vi "Accumulate data.vi"(6 "block size":i32, 9 "reset":bool, 10 "zero":bool, 11 "Accelerometer Data":T1={"Accel"=[0.0, 0.0, 0.0], "Gyro"=[0.0, 0.0, 0.0], "Time"=0, "Trigger"=FALSE}) -> (1 "done":bool, 2 "number in block":i32, 3 "Accelerometer Data Block":T2)   [LabVIEW 2013]
uses:
  I2C/Accelerometer Data Block.ctl
  I2C/Accelerometer Data.ctl
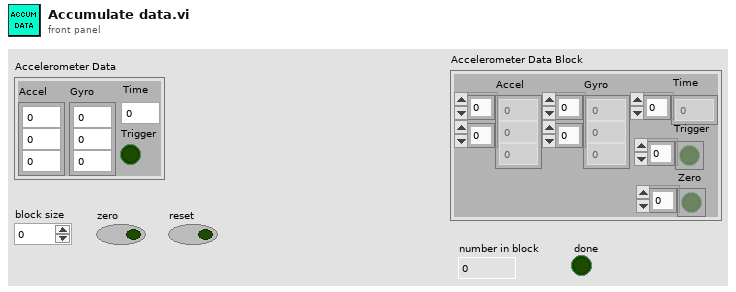
[diagram p1: front panel]
types:
  T1 = typedef "Accelerometer Data.ctl" = cluster{"Accel":dbl[], "Gyro":dbl[], "Time":u64, "Trigger":bool}
  T2 = typedef "Accelerometer Data Block.ctl" = cluster{"Accel":dbl[][], "Gyro":dbl[][], "Time":u64[], "Trigger":bool[], "Zero":bool[]}
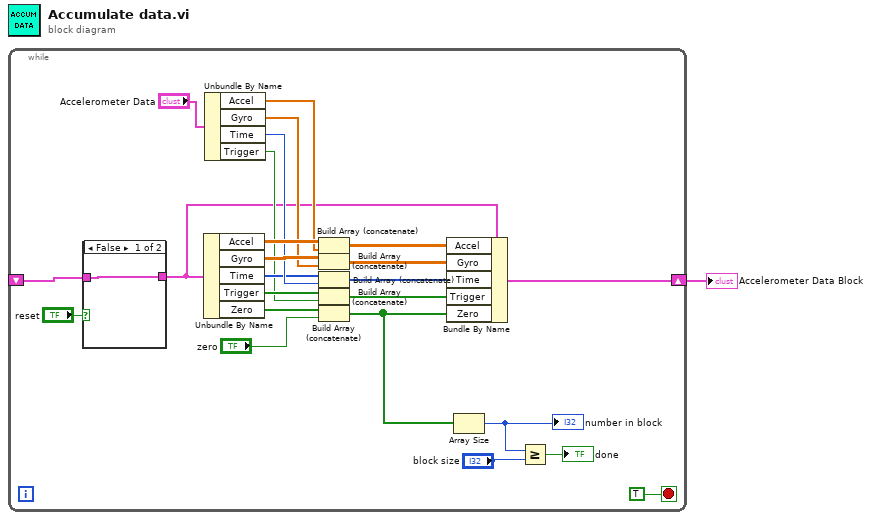
[diagram p0: block diagram]
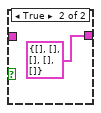
[diagram p2: hidden frame]
diagram:
  n1 = while {
    shift-right: [w4] -> w1
    shift-left: _ -> [w5]
    stop <- TRUE stop-if-true
    n2 = case shown="False" "reset" {
      tunnel: [w26 T2 {"Accel"=[], "Gyro"=[], "Time"=[], "Trigger"=[], "Zero"=[]} ("Accelerometer Data Block")] -> w3
      tunnel: w5 -> [w26 _]
      frame False {
      }
      frame True {
      }
    }
    n3 = Unbundle By Name(w3) -> ("Accel"=w24:dbl[][], "Gyro"=w23:dbl[][], "Time"=w21:u64[], "Trigger"=w20:bool[], "Zero"=w19:bool[])
    n4 = Unbundle By Name("Accelerometer Data") -> ("Accel"=w17:dbl[], "Gyro"=w16:dbl[], "Time"=w22:u64, "Trigger"=w15:bool)
    n5 = Build Array (concatenate)(w24, w17) -> (w14:dbl[][])
    n6 = Build Array (concatenate)(w23, w16) -> (w13:dbl[][])
    n7 = Build Array (concatenate)(w21, w22) -> (w12:u64[])
    n8 = Build Array (concatenate)(w20, w15) -> (w11:bool[])
    n9 = Build Array (concatenate)(w19, "zero") -> (w10:bool[])
    n10 = Bundle By Name(cluster=w3, "Accel"=w14, "Gyro"=w13, "Time"=w12, "Trigger"=w11, "Zero"=w10) -> (w4:T2)
    n11 = Array Size(array=w10) -> (size(s)=w9:i32)
    "number in block" <- w9
    n12 = Greater Or Equal?(x=w9, y="block size") -> (x >= y?=→"done":bool)
  }
  "Accelerometer Data Block" <- w1
